vi "Format Mapping Error.vi"(8 "error in (no error)":errorcluster, 11 "Type":T1) -> (0 "error out":errorcluster, 1 "mapping error out":errorcluster, 2 "mapping error name":string)   [LabVIEW 2020, in "Modbus Master System Explorer.lvlib"]
uses:
  Modbus Master System Explorer.lvlib
  Modbus Type.ctl
  Shared/Modbus Master Shared.lvlib
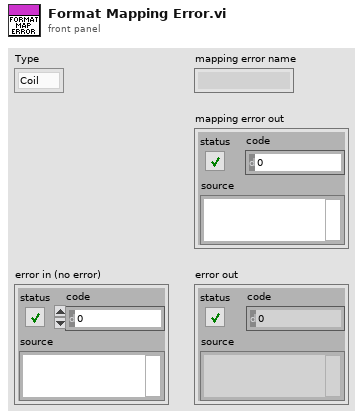
[diagram p1: front panel]
types:
  T1 = typedef "Modbus Master Shared.lvlib/Modbus Type.ctl" = enum16{"Coil", "Discrete Input", "Holding Register", "Input Register"}
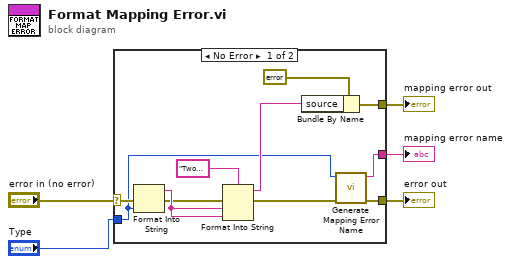
[diagram p0: block diagram]
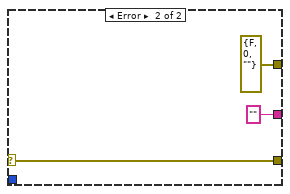
[diagram p2: hidden frame]
diagram:
  n1 = case shown="No Error" "error in (no error)" {
    selector: "error in (no error)" -> [w11 w19]
    tunnel: [w16 errorcluster {"status"=FALSE, "code"=0, "source"=""} ("error constant")] -> w5
    tunnel: [w8 w19] -> w3
    tunnel: [w7 "" ("String")] -> w2
    tunnel: "Type" -> [w6 _]
    frame No Error {
      n2 = Format Into String(error in=w11, w6) -> (resulting string=w12:string, error out=w10:errorcluster)  [unwired: 2 in]
      n3 = Format Into String(format string="Two %s channels are mapped to the same register. You can review conflicts on the \"%ss\" Group Settings Page.", error in=w10, w12, w12) -> (resulting string=w15:string, error out=w9:errorcluster)  [unwired: 1 in]
      n4 = Bundle By Name(cluster=errorcluster {"status"=TRUE, "code"=1000, "source"=""} ("error constant"), "source"=w15) -> (w16:errorcluster)
      n5 = call "Generate Mapping Error Name.vi"("error in"=w9, "Type"=w6) -> ("error out"=w8:errorcluster, "String"=w7:string)  [unwired: 8 in]
    }
    frame Error {
    }
  }
  "mapping error out" <- w5
  "error out" <- w3
  "mapping error name" <- w2
